vi "ModbusRequest.vi"(1 "ModbusSubnetTimestampFIFO":refnum<k21>="ModbusSubnetETxTimestampFIFO", 2 "ModbusSubnetRxFIFO":refnum<k21>="ModbusSubnetERxDataFIFO") -> ()   [LabVIEW 2016]
uses:
  <vilib>/rvi/DataTransferAndStorage/Container/Common/niFpgaContainerExecOnDevCompGetState.vi
  <vilib>/rvi/Emulation/niFpgaEmulationIsFPGAContextNoSignature.vi
  <vilib>/rvi/Emulation/niFpgaSctlEmulationGetInTimedLoop.vi
  <vilib>/rvi/errors/niFpgaSetErrorForExecOnDevCompSimple.vi
  <vilib>/rvi/eio/common/nirviEmuReportErrorAndStop.vi
  <vilib>/rvi/DataTransferAndStorage/Container/Common/niFpgaContainerGetUniqueNameForEmu.vi
  <vilib>/rvi/FIFO/Fifo_Resource/nirvififoEmulationSetSize.vi
  <vilib>/rvi/FIFO/Fifo_Resource/nirviFifoEmulationQueueMgr.vi
  <instcachedir>/0/nirviFifoEmulationQueueMgr_E5CAEC123FF24DC58D834DCA3CDAA9B5.lvgen/nirviFifoEmulationQueueMgr_E5CAEC123FF24DC58D834DCA3CDAA9B5_002.vi
  <vilib>/rvi/FIFO/Fifo_Resource/nirvififoEmulationDetermineInputValidOut.vi
  <vilib>/rvi/FIFO/Fifo_Resource/nirvififoEmulationCreateLock.vi
  <vilib>/rvi/Emulation/niFpgaProcessEmulError.vi
  <vilib>/rvi/FIFO/Fifo_Resource/nirvififoEmulationObtainLock.vi
  <vilib>/rvi/FIFO/Fifo_Resource/nirvififoEmulationReleaseLock.vi
  <vilib>/rvi/occurrence/nirviWaitOnOccurrenceBase.vi
  <vilib>/rvi/errors/nirviReportUnexpectedCaseInternalError.vi
  <vilib>/rvi/errors/nirviReportUnexpectedCaseInternalError (U32).vi
  <vilib>/Utility/error.llb/Clear Errors.vi
  <vilib>/rvi/interface/RandomDataEmulation/niFpgaRandomDataHandleErrors.vi
  <instcachedir>/0/nirviFifoEmulationQueueMgr_E5CAEC123FF24DC58D834DCA3CDAA9B5.lvgen/nirviFifoEmulationQueueMgr_E5CAEC123FF24DC58D834DCA3CDAA9B5_007.vi
  <vilib>/rvi/DataTransferAndStorage/Container/XNode/niFpgaContainer.xnode
  <vilib>/rvi/FIFO/Fifo_Resource/niFpgaFifoEmulationRefIn.vi
  <vilib>/rvi/interface/RandomDataEmulation/nirviRandomDataFpgaReadWriteTemplate.vi
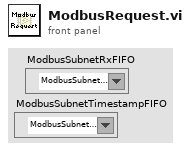
[diagram p1: front panel]
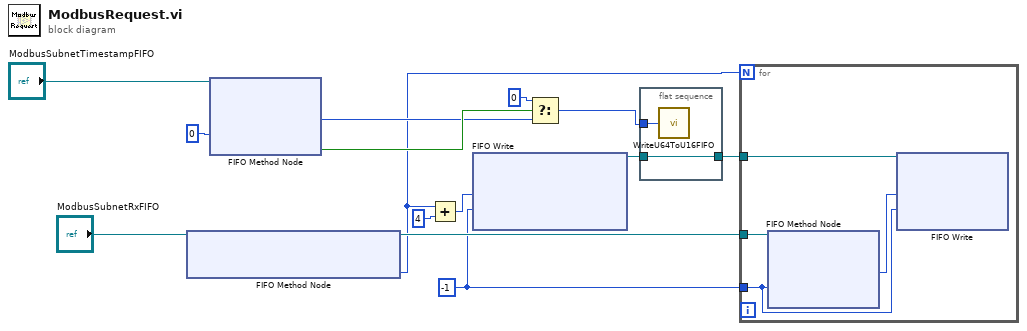
[diagram p0: block diagram]
diagram:
  w13 = -1 ("Timeout")
  n1 = xnode ("FIFO Method Node")("FIFO In"="ModbusSubnetRxFIFO") -> ("Number of Elements to Read"=w6:u32, "FIFO Out"=w14:refnum<k21>)
  n2 = xnode ("FIFO Method Node")("Timeout"=0, "FIFO In"="ModbusSubnetTimestampFIFO") -> ("Element"=w8:u64, "Timed Out?"=w9:bool)  [unwired: 1 out]
  n3 = Add(x=w6, y=u32 4) -> (x+y=w4:u32)
  n4 = xnode ("FIFO Write")("Element"=w4, "Timeout"=w13) -> ("FIFO Out"=w1:refnum<k21>)  [unwired: 1 in, 1 out]
  n5 = Select(t=u64 0, s=w9, f=w8) -> (s? t:f=w3:u64)
  n6 = flat-sequence {
    tunnel: w3 -> [w16]
    tunnel: [w15] -> w2
    tunnel: w1 -> [w15]
    frame #0 {
      n7 = call "WriteU64ToU16FIFO.vi"("U64"=w16) -> ()  [unwired: 1 in]
    }
  }
  n8 = for {
    N: w6 -> [_]
    tunnel: w14 -> [w20]
    tunnel: w2 -> [w19]
    tunnel: w13 -> [w18]
    n9 = xnode ("FIFO Method Node")("Timeout"=w18, "FIFO In"=w20) -> ("Element"=w17:u16)  [unwired: 2 out]
    n10 = xnode ("FIFO Write")("Element"=w17, "Timeout"=w18, "FIFO In"=w19) -> ()  [unwired: 2 out]
  }
